vi "Configure Voltage (High Voltage).vi"(8 "error in (no error)":errorcluster, 10 "High Voltage (1.00 V)":dbl=1.0, 11 "VISA resource name":refnum<visa-resource-name>) -> (0 "error out":errorcluster, 3 "VISA resource name out":refnum<visa-resource-name>)   [LabVIEW 2017, in "Keithley 3390.lvlib"]
doc: "Configures the High voltage of the currently active waveform.\n\n<b>Notes:</b>\nSpecifying a high voltage level and a low level voltage is equivlent to specifying amplitude and DC offset. For example, if you set the high level to +2 volts and the low level to -3 volts, the resulting amplitude will be 5 Vpp, with DC offset at -0.5 V."
uses:
  Keithley 3390.lvlib
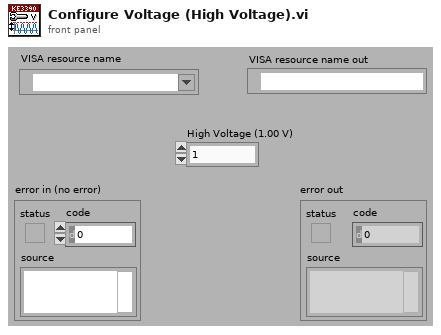
[diagram p1: front panel]
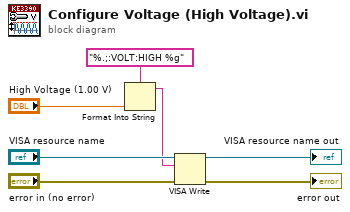
[diagram p0: block diagram]
diagram:
  n1 = Format Into String(format string="%.;:VOLT:HIGH %g", "High Voltage (1.00 V)") -> (resulting string=w4:string)  [unwired: 2 in, 1 out]
  n2 = VISA Write(VISA resource name="VISA resource name", write buffer=w4, error in (no error)="error in (no error)") -> (VISA resource name out=→"VISA resource name out":refnum<visa-resource-name>, error out=→"error out":errorcluster)  [unwired: 1 out]
